vi "drive straight - dad cop 2.vi"(2 "Reverse":bool, 3 "Speed":dbl) -> (0 "right":dbl, 1 "left":dbl)   [LabVIEW 2011]
uses:
  Robot Global Data.vi
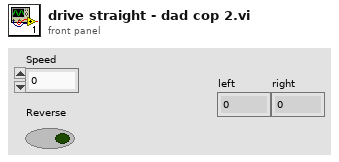
[diagram p1: front panel]
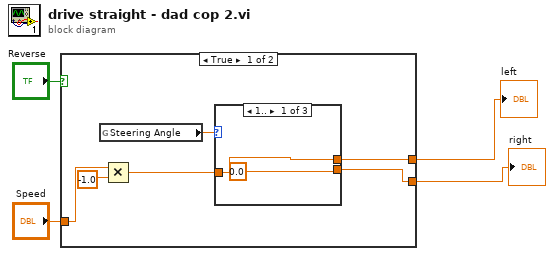
[diagram p0: block diagram]
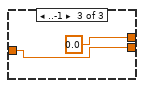
[diagram p3: hidden frame]
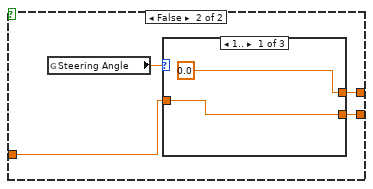
[diagram p4: hidden frame]
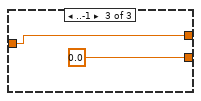
[diagram p6: hidden frame]
diagram:
  n1 = case shown="True" "Reverse" {
    tunnel: "Speed" -> [w9 w18]
    tunnel: [w6 w17] -> w2
    tunnel: [w5 w16] -> w1
    frame True {
      n2 = global read "Robot Global Data.vi" "Steering Angle"() -> (w10:dbl)
      n3 = Multiply(x=w9, y=-1.0) -> (x*y=w7:dbl)
      n4 = case shown="1.." w10 {
        tunnel: w7 -> [w11 w13 w14]
        tunnel: [w11 w13 0.0 ("X axis value")] -> w6
        tunnel: [0.0 ("X axis value") w13 w14] -> w5
        frame 1.. {
        }
        frame Default {
        }
        frame ..-1 {
        }
      }
    }
    frame False {
      n5 = global read "Robot Global Data.vi" "Steering Angle"() -> (w19:dbl)
      n6 = case shown="1.." w19 {
        tunnel: w18 -> [w20 w22 w24]
        tunnel: [0.0 ("X axis value") w22 w24] -> w17
        tunnel: [w20 w22 0.0 ("Right axis value")] -> w16
        frame 1.. {
        }
        frame Default {
        }
        frame ..-1 {
        }
      }
    }
  }
  "left" <- w2
  "right" <- w1
